vi "ROS_Master_nodeFromPubSub.vi"(2 "PubSub":T2) -> (0 "Node":T1)   [LabVIEW 2012]
doc: "Returns the node for a given publisher or subscriber"
uses:
  <userlib>/ROSforLV/ROS/Code/ROS_Master/ROS_Topic.ctl
  <userlib>/ROSforLV/ROS/Code/ROS_Master/ROS_Node.ctl
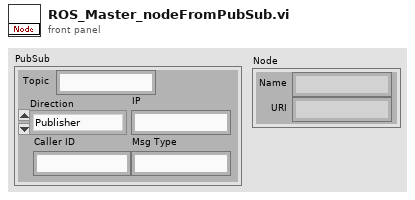
[diagram p1: front panel]
types:
  T1 = typedef "ROS_Node.ctl" = cluster{"Name":string, "URI":string}
  T2 = typedef "ROS_Topic.ctl" = cluster{"Caller ID":string, "IP":string, "Msg Type":string, "Direction":enum16{"Publisher", "Subscriber"}, "Topic":string}
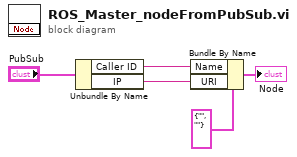
[diagram p0: block diagram]
diagram:
  n1 = Unbundle By Name("PubSub") -> ("Caller ID"=w4:string, "IP"=w3:string)
  n2 = Bundle By Name(cluster=T1 {"Name"="", "URI"=""} ("Node"), "Name"=w4, "URI"=w3) -> (→"Node":T1)
